vi "Read Subsystem Configuration.vi"(8 "error in (no error)":errorcluster, 11 "Configuration Refnum In":T2) -> (0 "error out":errorcluster, 2 "Subsystems":T1[](array[typedef]), 3 "Configuration Refnum Out":T2)   [LabVIEW 2024]
doc: "Reads the subsystem configurations."
uses:
  <vilib>/Utility/config.llb/Config Data RefNum.ctl
  Controls/Server/Subsystem Configuration.ctl
  <vilib>/Utility/config.llb/Read Key (String).vi
  <vilib>/Utility/config.llb/NI_LVConfig.lvlib
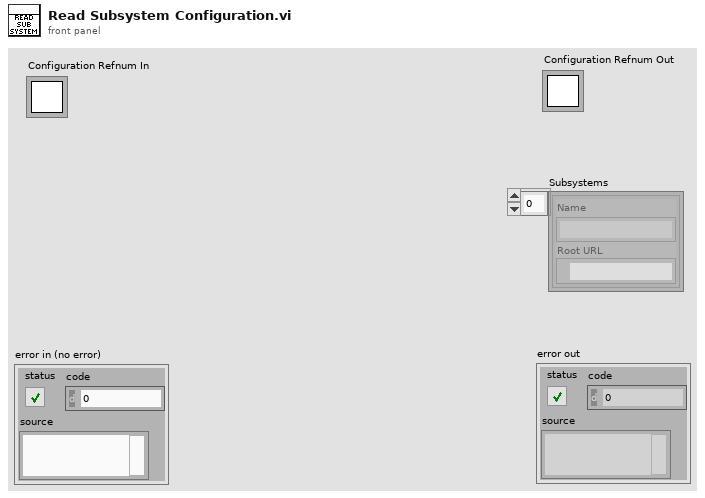
[diagram p1: front panel]
types:
  T1 = typedef "Subsystem Configuration.ctl" = cluster{"Name":string, "Root URL":refnum<k21>}
  T2 = typedef "NI_LVConfig.lvlib/Config Data RefNum.ctl" = refnum<k1>
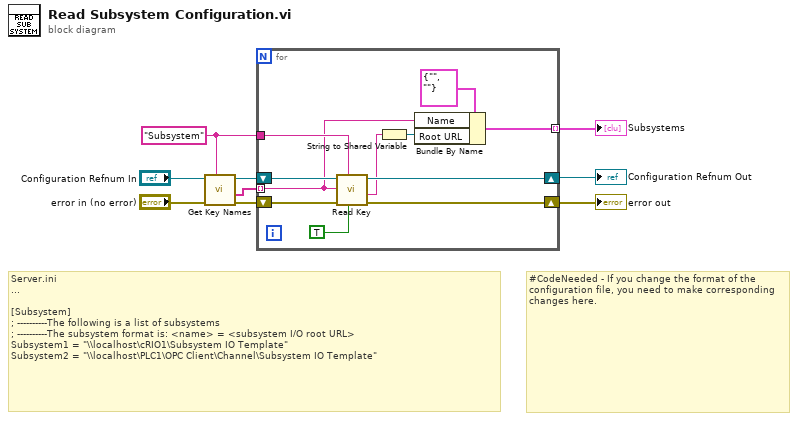
[diagram p0: block diagram]
diagram:
  w2 = "Subsystem" ("section")
  # "#CodeNeeded - If you change the format of the configuration file, you need to make corresponding changes here."
  # "Server.ini\n...\n\n[Subsystem]\n; ----------The following is a list of subsystems\n; ----------The subsystem format is: <name> = <subsystem I/O root URL>\nSubsystem1 = \"\\\\localhost\\cRIO1\\Subsystem IO Template\"\nSubsystem2 = \"\\\\localhost\\PLC1\\OPC Client\\Channel\\Subsystem IO Template\""
  n1 = call <vilib>:"Get Key Names.vi"("section"=w2, "error in (no error)"="error in (no error)", "refnum"="Configuration Refnum In") -> ("error out"=w4:errorcluster, "key names"=w8:string[], "refnum out"=w7:T2)  [unwired: 5 in, 1 out]
  n2 = for {
    tunnel: w8 -> [w16] mode=indexing
    shift-right: [w15] -> w6
    shift-left: w7 -> [w19]
    shift-right: [w14] -> w3
    shift-left: w4 -> [w18]
    tunnel: w2 -> [w20]
    tunnel: [w10] -> w1 mode=indexing
    n3 = call-poly <vilib>:"Read Key.vi"("read raw string? (F)"=TRUE, "section"=w20, "error in (no error)"=w18, "key"=w16, "refnum"=w19) -> ("error out"=w14:errorcluster, "value"=w13:string, "refnum out"=w15:T2)  [unwired: 3 in, 1 out]
    n4 = String to Shared Variable(0:w13) -> (2:w12:refnum<k21>)  [unwired: 1 out]
    n5 = Bundle By Name(cluster=T1 {"Name"="", "Root URL"=""} ("Subsystem"), "Name"=w16, "Root URL"=w12) -> (w10:T1)
  }
  "error out" <- w3
  "Configuration Refnum Out" <- w6
  "Subsystems" <- w1
